vi "HapticSTM_rawspeed.vi"() -> ()   [LabVIEW 2019]
uses:
  SubVIs/GlobalClicksHeight_raw.vi
  <userlib>/HapticSTM/HapticSTM.lvlib
  <userlib>/Nanonis Prog Interface V5/Nanonis Prog Interface.lvlib
panel:
  in  "Z Write?":bool
  in  "Save":bool
  in  "# Sample Points":i32=4096
  in  "Depth (pA)":dbl=280.0
  in  "Shift (in)":dbl format="%.1f"
  in  "Hardness":dbl=0.7 format="%.1f"
  in  "Scaling?":u16(ring) items=["Medium", "Large", "Small"]
  out "Setpoint (pA)":dbl
  in  "Maximum (pA)":dbl=7000.0
  out "Filtered Current (pA)":dbl format="%.1f"
  out "Current (pA)":dbl format="%.1f"
  out "Oy":dbl
  out "Ox":dbl
  out "W":dbl
  out "H":dbl
  out "Z Write":dbl format="%^.1e"
  in  "Planing?":bool
  out "Fy":dbl format="%.1f"
  out "Fz":dbl format="%.1f"
  out "Fx":dbl format="%.1f"
  out "x":dbl format="%.1f"
  out "y":dbl format="%.1f"
  out "z":dbl format="%0.1f"
  in  "Mode":u16(ring) items=["Log w/ Exp Z", "Log w/ Lin Z", "Coulomb Force", "Lennard Jones", "r^6"]
  in  "Reset Clicks":bool
  out "Clicks":i32
  in  "STOP":bool
  in  "START":bool
  out "Raw and Scaled Z Positions":T1(graph)
  out "Scaled Force and Current":T2(graph)
  # "Super Ultra Mega Haptic STM Controller 3000"
  # "Haptic Pen"
  # "Nanonis"
  # "Position"
  # "Z Controller"
  # "Force"
  # "Frame"
  # "Surface"
  # "Options"
  # "Addons"
  # "Current"
  # "No"
  # "Yes"
  # "Planing"
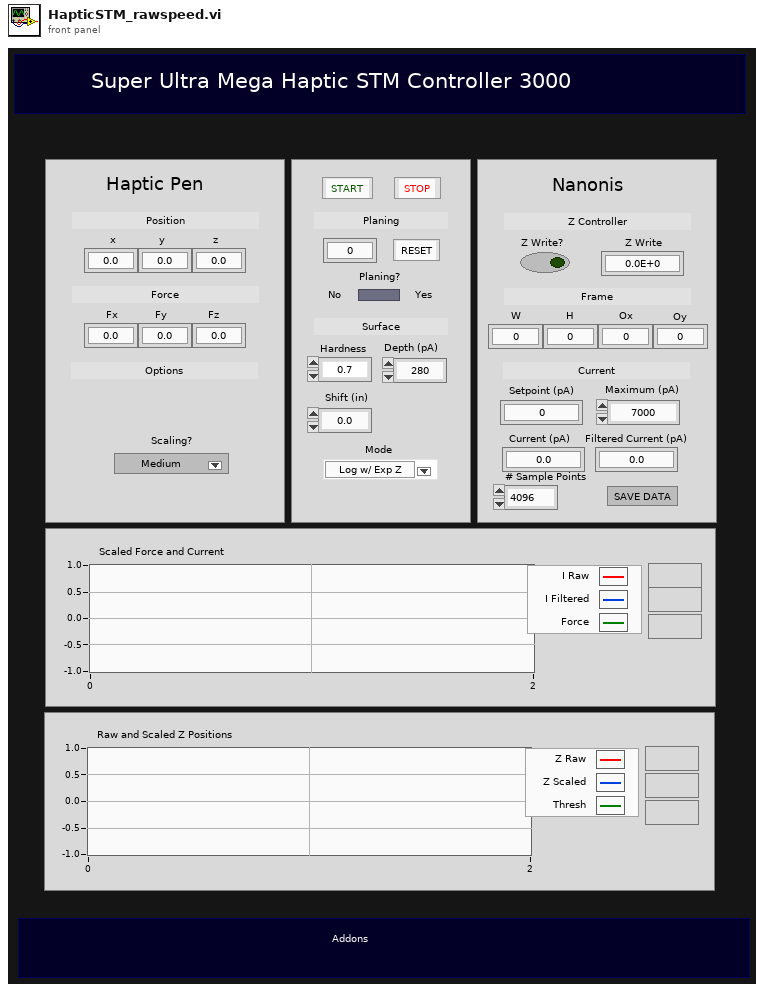
[diagram p1: front panel]
types:
  T1 = cluster{dbl, "function return":dbl, "function return":dbl}
  T2 = cluster{"Current (pA)":dbl, "Filtered Current (pA)":dbl, dbl}
  T3 = cluster{"Size (m)":cluster{"Width":sgl, "Height":sgl}, "Center coordinates (m)":cluster{"Xc":sgl, "Yc":sgl}}
  T4 = cluster{"Z Raw":dbl, "Z scaled":dbl, "threshhold":dbl}
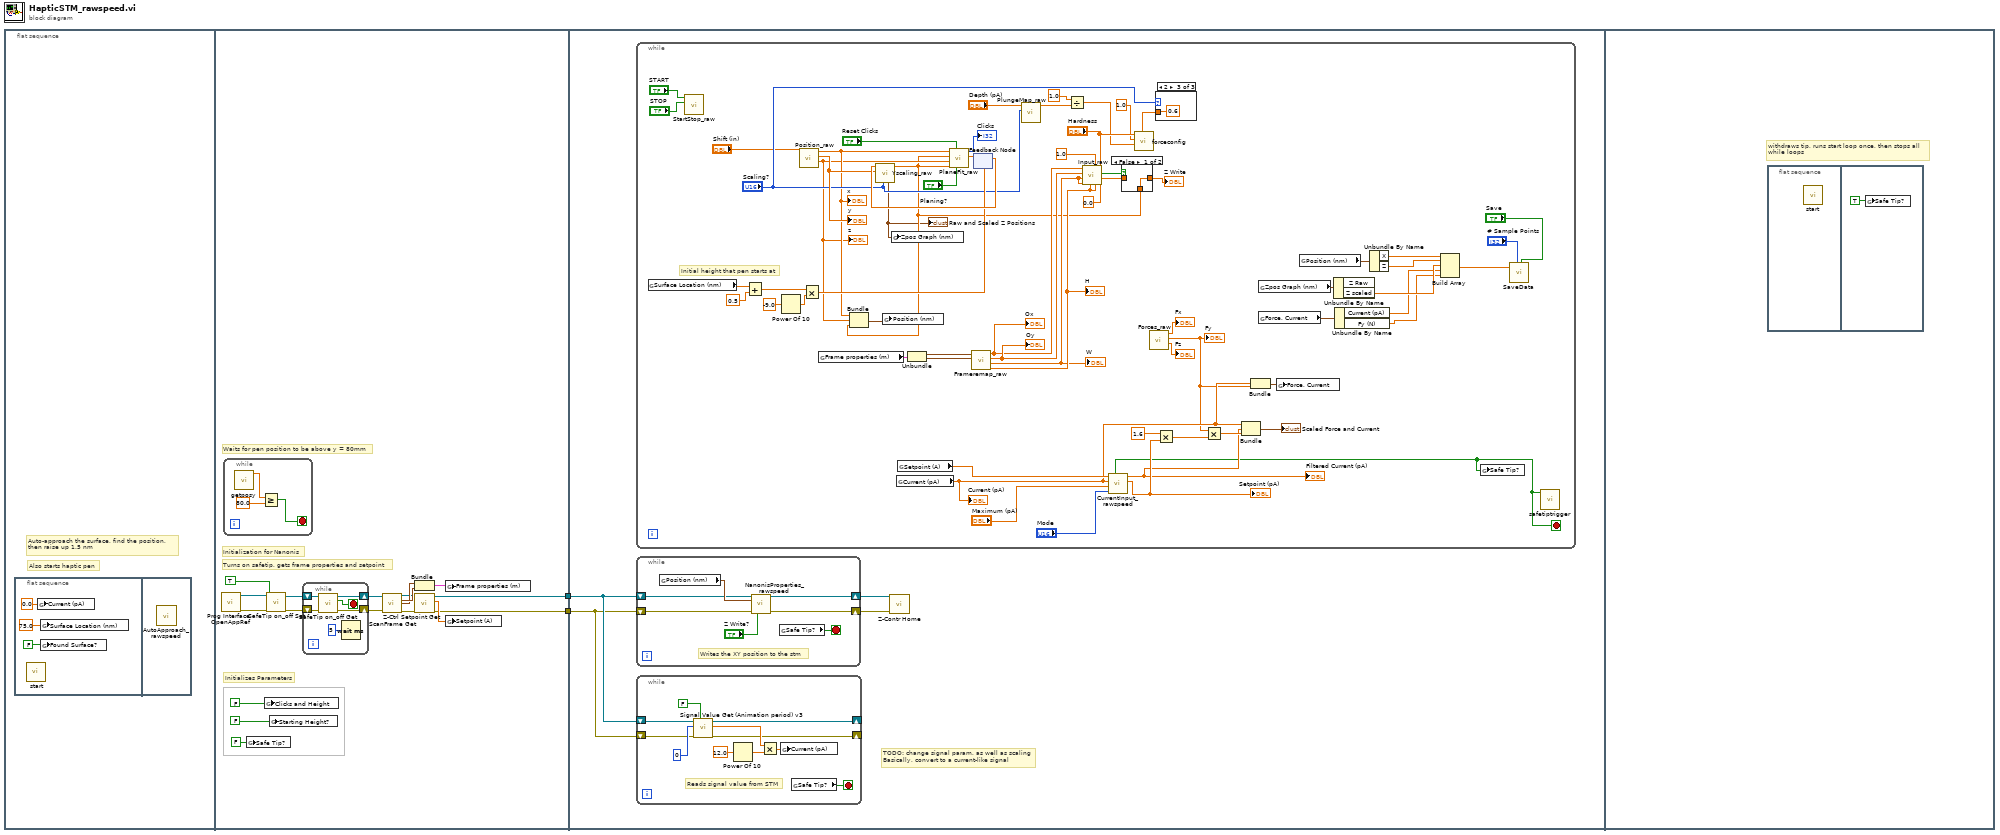
[diagram p0: block diagram]
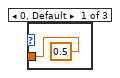
[diagram p2: hidden frame]
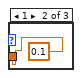
[diagram p3: hidden frame]
diagram:
  n1 = flat-sequence {
    tunnel: [w7] -> w2
    tunnel: [w6] -> w1
    tunnel: w2 -> [w36]
    tunnel: w1 -> [w35]
    frame #0 {
      # "Also starts haptic pen"
      # "Auto-approach the surface, find the position, \nthen raise up 1.5 nm"
      n2 = flat-sequence {
        frame #0 {
          n3 = call <userlib>:"start.vi"() -> ()  [unwired: 11 in, 1 out]
          n4 = global write "GlobalClicksHeight_raw.vi" "Current (pA)"(0.0 ("Current (pA)")) -> ()
          n5 = global write "GlobalClicksHeight_raw.vi" "Surface Location (nm)"(75.0 ("Surface Location")) -> ()
          n6 = global write "GlobalClicksHeight_raw.vi" "Found Surface?"(FALSE ("Clicks and Height")) -> ()
        }
        frame #1 {
          n7 = call "AutoApproach_rawspeed.vi"() -> ()  [unwired: 12 in]
        }
      }
    }
    frame #1 {
      # "Turns on safetip, gets frame properties and setpoint"
      # "Waits for pen position to be above y = 80mm"
      # "Initializes Parameters"
      # "Initialization for Nanonis"
      n8 = call <userlib>:"Prog Interface - OpenAppRef.vi"() -> ("Error out"=w13:errorcluster, "Application reference"=w12:refnum<vi>)  [unwired: 6 in]
      n9 = while {
        stop <- w24 stop-if-true
        n10 = call <userlib>:"getposy.vi"() -> ("function return"=w26:dbl)  [unwired: 11 in]
        n11 = Greater Or Equal?(x=w26, y=80.0) -> (x >= y?=w24:bool)
      }
      n12 = global write "GlobalClicksHeight_raw.vi" "Safe Tip?"(FALSE ("Safe Tip?")) -> ()
      n13 = global write "GlobalClicksHeight_raw.vi" "Clicks and Height"(FALSE ("Clicks and Height")) -> ()
      n14 = call <userlib>:"SafeTip on_off Set.vi"("error in (no error)"=w13, "SafeTip ON/OFF"=TRUE, "Application ref in"=w12) -> ("error out"=w15:errorcluster, "Application ref out"=w14:refnum<vi>)  [unwired: 7 in]
      n15 = global write "GlobalClicksHeight_raw.vi" "Starting Height?"(FALSE ("Clicks and Height")) -> ()
      n16 = while {
        shift-right: [w29] -> w16
        shift-left: w14 -> [w31]
        shift-right: [w28] -> w17
        shift-left: w15 -> [w30]
        stop <- w32 stop-if-true
        n17 = call <userlib>:"SafeTip on_off Get.vi"("error in (no error)"=w30, "Application ref in"=w31) -> ("error out"=w28:errorcluster, "SafeTip on/off status"=w32:bool, "Application ref out"=w29:refnum<vi>)  [unwired: 7 in]
        n18 = Wait (ms)(milliseconds to wait=u32 5) -> ()  [unwired: 1 out]
      }
      n19 = call <userlib>:"ScanFrame Get.vi"("Application ref in"=w16, "error in (no error)"=w17) -> ("Application ref out"=w18:refnum<vi>, "Center coordinates (m)"=w23:cluster{"Xc":sgl, "Yc":sgl}, "Size (m)"=w22:cluster{"Width":sgl, "Height":sgl}, "error out"=w19:errorcluster)  [unwired: 9 in, 1 out]
      n20 = Bundle("Size (m)"=w22, "Center coordinates (m)"=w23) -> (w21:T3)  [unwired: 1 in]
      n21 = call <userlib>:"Z-Ctrl Setpoint Get.vi"("error in (no error)"=w19, "Application ref in"=w18) -> ("error out"=w6:errorcluster, "Z Controller setpoint"=w20:sgl, "Application ref out"=w7:refnum<vi>)  [unwired: 6 in]
      n22 = global write "GlobalClicksHeight_raw.vi" "Frame properties (m)"(w21) -> ()
      n23 = global write "GlobalClicksHeight_raw.vi" "Setpoint (A)"(w20) -> ()
    }
    frame #2 {
      # "TODO: change signal param, as well as scaling\nBasically, convert to a current-like signal"
      n24 = while {
        stop <- w55 stop-if-true
        # "Initial height that pen starts at"
        n25 = global read "GlobalClicksHeight_raw.vi" "Surface Location (nm)"() -> (w78:dbl)
        n26 = call "StartStop_raw.vi"("STOP"="STOP", "START"="START") -> ()  [unwired: 10 in]
        n27 = Add(x=w78, y=0.5) -> (x+y=w75:dbl)
        n28 = Power Of 10(x=-9.0) -> (10^x=w74:dbl)
        n29 = call "Position_raw.vi"("Shift"="Shift (in)") -> ("Z"=w67:dbl, "Y"=w99:dbl, "X"=w68:dbl)  [unwired: 8 in]
        "x" <- w68
        "y" <- w99
        "z" <- w67
        n30 = Multiply(x=w75, y=w74) -> (x*y=w76:dbl)
        n31 = global read "GlobalClicksHeight_raw.vi" "Frame properties (m)"() -> (w64:cluster{cluster{dbl, dbl}, cluster{dbl, dbl}})
        n32 = global read "GlobalClicksHeight_raw.vi" "Current (pA)"() -> (w59:dbl)
        "Current (pA)" <- w59
        n33 = global read "GlobalClicksHeight_raw.vi" "Setpoint (A)"() -> (w65:dbl)
        n34 = Unbundle(w64) -> (w63:cluster{dbl, dbl}, w62:cluster{dbl, dbl})
        n35 = call "Frameremap_raw.vi"("Frame Origin (m)"=w62, "Frame Size (m)"=w63) -> ("FH (nm)"=w88:dbl, "FW (nm)"=w87:dbl, "Z Origin (nm)"=w86:dbl, "X Origin (nm)"=w85:dbl)  [unwired: 6 in]
        "H" <- w88
        "W" <- w87
        "Ox" <- w85
        "Oy" <- w86
        n36 = feedback #1(w76) -> (w103:dbl)
        n37 = call "Yscaling_raw.vi"("Scaling?"="Scaling?", "Y"=w99, "Plane Height (m)"=w103) -> ("y scaled (m)"=w66:dbl, "Zpos Graph (nm)"=w57:T1)  [unwired: 7 in]
        "Raw and Scaled Z Positions" <- w57
        n38 = Bundle("X"=w68, "Z"=w67, "y scaled (m)"=w66) -> (w69:cluster{"X":dbl, "Z":dbl, "y scaled (m)":dbl})  [unwired: 1 in]
        n39 = global write "GlobalClicksHeight_raw.vi" "Position (nm)"(w69) -> ()
        n40 = global write "GlobalClicksHeight_raw.vi" "Zpos Graph (nm)"(w57) -> ()
        n41 = call "PlaneFit_raw.vi"("Planing y/n?"="Planing?", "Reset Clicks"="Reset Clicks", "Y PEN"=w66, "Z"=w67, "Nano Z"=w66, "X"=w68) -> ("Plane Height (m)"=w104:dbl, "Clicks"=→"Clicks":i32)  [unwired: 3 in, 1 out]
        n42 = feedback-in #1(w104) -> ()
        n43 = call "PlungeMap_raw.vi"("Scaling?"="Scaling?", "Input (pA)"="Depth (pA)") -> ("output"=w79:dbl)  [unwired: 9 in]
        n44 = Divide(x=1.0, y=w79) -> (x/y=w89:dbl)
        n45 = call "Input_raw.vi"("Current * 10^input"=0.0, "Sensitivity"="Hardness", "Scopez"=w88, "Drag"=1.0, "FH"=w88, "FW"=w87, "Scopex"=w87, "Z origin"=w86, "X origin"=w85) -> ("Scaled Current"=w91:dbl, "feedback"=w93:bool)  [unwired: 1 in]
        n46 = call "CurrentInput_rawspeed.vi"("Mode"="Mode", "Maximum (pA)"="Maximum (pA)", "Current (pA)"=w59, "Setpoint (A)"=w65) -> ("Setpoint (pA)"=w81:dbl, "Filtered Current (pA)"=w58:dbl, "Safetip?"=w55:bool)  [unwired: 5 in]
        "Filtered Current (pA)" <- w58
        "Setpoint (pA)" <- w81
        n47 = case shown="False" w93 {
          tunnel: [w124 w125] -> w92
          tunnel: w91 -> [_ w125]
          tunnel: w66 -> [w124 _]
          frame False {
          }
          frame True {
          }
        }
        "Z Write" <- w92
        n48 = call "Forces_raw.vi"() -> ("Fz"=→"Fz":dbl, "Fy"=w56:dbl, "Fx"=→"Fx":dbl)  [unwired: 9 in]
        "Fy" <- w56
        n49 = case shown="2" "Scaling?" {
          tunnel: [0.5 0.1 0.6] -> w72
          frame 0, Default {
          }
          frame 1 {
          }
          frame 2 {
          }
        }
        n50 = call <userlib>:"forceconfig.vi"("spc"=w72, "c"=w89, "b"=1.0, "a"="Hardness") -> ()  [unwired: 8 in]
        n51 = Multiply(x=1.6 ("y"), y=w81) -> (x*y=w100:dbl)
        n52 = Multiply(x=w56, y=w100) -> (x*y=w102:dbl)
        n53 = Bundle("Current (pA)"=w59, "Filtered Current (pA)"=w58, w102) -> (→"Scaled Force and Current":T2)  [unwired: 1 in]
        n54 = Bundle("Current (pA)"=w59, "Fy"=w56) -> (w60:cluster{"Current (pA)":dbl, "Fy":dbl})  [unwired: 1 in]
        n55 = global read "GlobalClicksHeight_raw.vi" "Force, Current"() -> (w115:cluster{"Current (pA)":dbl, "Fy (N)":dbl})
        n56 = global read "GlobalClicksHeight_raw.vi" "Zpos Graph (nm)"() -> (w117:T4)
        n57 = global write "GlobalClicksHeight_raw.vi" "Force, Current"(w60) -> ()
        n58 = global read "GlobalClicksHeight_raw.vi" "Position (nm)"() -> (w120:cluster{"X":dbl, "Z":dbl, "Y":dbl})
        n59 = Unbundle By Name(w117) -> ("Z scaled"=w116:dbl)  [unwired: 1 out]
        n60 = Unbundle By Name(w115) -> ("Current (pA)"=w114:dbl, "Fy (N)"=w113:dbl)
        n61 = Unbundle By Name(w120) -> ("X"=w119:dbl, "Z"=w118:dbl)
        n62 = Build Array(w119, w118, w116, w114, w113) -> (w112:dbl[])
        n63 = global write "GlobalClicksHeight_raw.vi" "Safe Tip?"(w55) -> ()
        n64 = call "SaveData.vi"("Save"="Save", "# Sample Points"="# Sample Points", "Data"=w112) -> ()  [unwired: 9 in]
        n65 = call <userlib>:"safetiptrigger.vi"("triggered"=w55) -> ()  [unwired: 11 in]
      }
      n66 = while {
        shift-right: [w48] -> w33
        shift-left: w35 -> [w50]
        shift-right: [w49] -> w34
        shift-left: w36 -> [w51]
        stop <- w54 stop-if-true
        # "Writes the XY position to the stm"
        n67 = global read "GlobalClicksHeight_raw.vi" "Position (nm)"() -> (w52:cluster{"X":dbl, "Z":dbl, "Y":dbl})
        n68 = call "NanonisProperties_rawspeed.vi"("Application ref in"=w51, "Position (nm)"=w52, "error in (no error)"=w50, "Z Write?"="Z Write?") -> ("Application ref out"=w49:refnum<vi>, "error out"=w48:errorcluster)  [unwired: 10 in]
        n69 = global read "GlobalClicksHeight_raw.vi" "Safe Tip?"() -> (w54:bool)
      }
      n70 = while {
        shift-right: [w39] -> _
        shift-left: w35 -> [w41]
        shift-right: [w40] -> _
        shift-left: w36 -> [w37]
        stop <- w47 stop-if-true
        # "Reads signal value from STM"
        n71 = call <userlib>:"Signal Value Get (Animation period) v3.vi"("Wait for newest data (F=False)"=FALSE, "error in (no error)"=w41, "Signal index (0-127)"=i8 0, "Application ref in"=w37) -> ("error out"=w39:errorcluster, "Signal value"=w42:sgl, "Application ref out"=w40:refnum<vi>)  [unwired: 4 in]
        n72 = Power Of 10(x=12.0) -> (10^x=w45:dbl)
        n73 = Multiply(x=w42, y=w45) -> (x*y=w44:dbl)
        n74 = global write "GlobalClicksHeight_raw.vi" "Current (pA)"(w44) -> ()
        n75 = global read "GlobalClicksHeight_raw.vi" "Safe Tip?"() -> (w47:bool)
      }
      n76 = call <userlib>:"Z-Contr Home.vi"("Error in (no error)"=w33, "Application ref in"=w34) -> ()  [unwired: 8 in, 2 out]
    }
    frame #3 {
      # "withdraws tip, runs start loop once, then stops all\nwhile loops"
      n77 = flat-sequence {
        frame #0 {
          n78 = call <userlib>:"start.vi"() -> ()  [unwired: 11 in, 1 out]
        }
        frame #1 {
          n79 = global write "GlobalClicksHeight_raw.vi" "Safe Tip?"(TRUE ("Safe Tip?")) -> ()
        }
      }
    }
  }
